vi "Real Moving Average testing.vi"() -> ()   [LabVIEW 2009]
panel:
  out "Waveform Graph":cluster{"Average Array":dbl[]}[](graph)
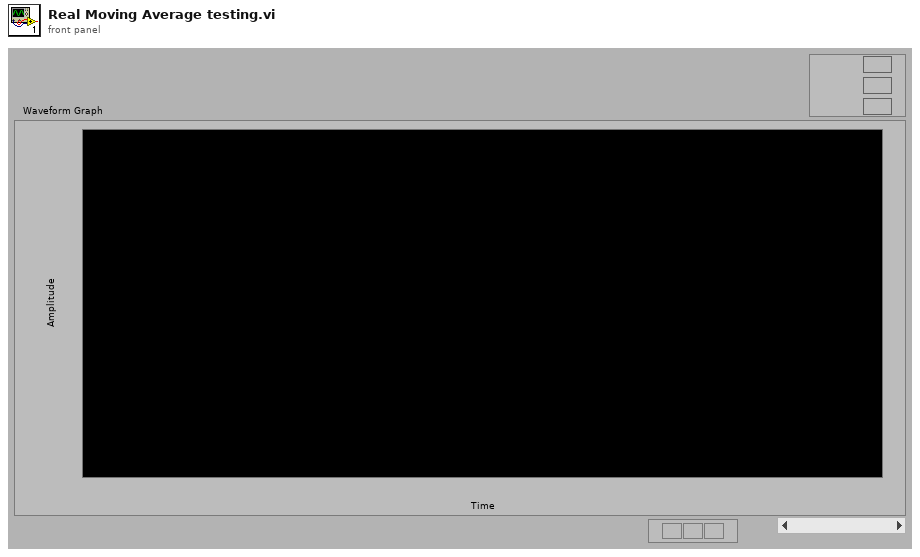
[diagram p1: front panel]
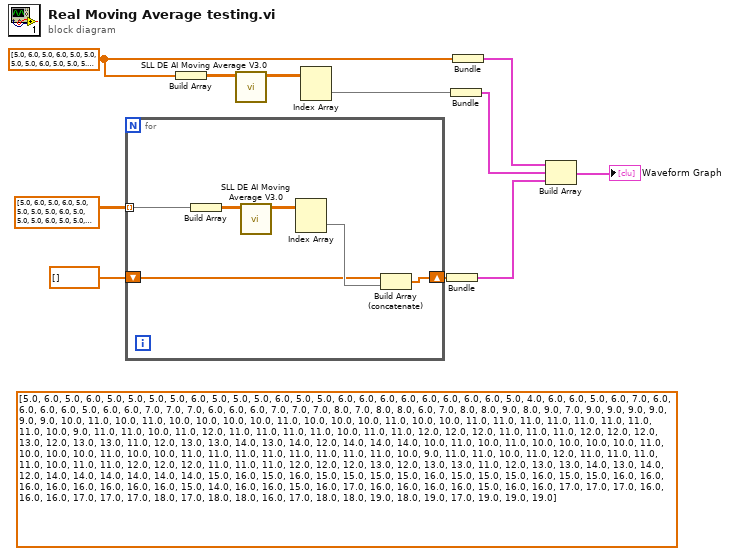
[diagram p0: block diagram]
diagram:
  (unwired) dbl[][] [[5.0, 6.0, 5.0, 6.0, 5.0, 5.0, 5.0, 5.0, 6.0, 5.0, 5.0, 5.0, 6.0, 5.0, 5.0, 6.0, 6.0, 6.0, 6.0, 6.0, 6.0, 6.0, 6.0, 5.0, 4.0, 6.0, 6.0, 5.0, 6.0, 7.0, 6.0, 6.0, 6.0, 6.0, 5.0, 6.0, 6.0, 7.0, 7.0, 7.0, 6.0, 6.0, 6.0, 7.0, 7.0, 7.0, 8.0, 7.0, 8.0, 8.0], [6.0, 7.0, 8.0, 8.0, 9.0, 8.0, 9.0, 7.0, 9.0, 9.0, 9.0, 9.0, 9.0, 9.0, 10.0, 11.0, 10.0, 11.0, 10.0, 10.0, 10.0, 10.0, 11.0, 10.0, 10.0, 10.0, 11.0, 10.0, 10.0, 11.0, 11.0, 11.0, 11.0, 11.0, 11.0, 11.0, 11.0, 10.0, 9.0, 11.0, 11.0, 10.0, 11.0, 12.0, 11.0, 11.0, 11.0, 11.0, 10.0, 11.0], [11.0, 12.0, 12.0, 12.0, 11.0, 11.0, 11.0, 12.0, 12.0, 12.0, 13.0, 12.0, 13.0, 13.0, 11.0, 12.0, 13.0, 13.0, 14.0, 13.0, 14.0, 12.0, 14.0, 14.0, 14.0, 10.0, 11.0, 10.0, 11.0, 10.0, 10.0, 10.0, 10.0, 11.0, 10.0, 10.0, 10.0, 11.0, 10.0, 10.0, 11.0, 11.0, 11.0, 11.0, 11.0, 11.0, 11.0, 11.0, 10.0, 9.0], [11.0, 11.0, 10.0, 11.0, 12.0, 11.0, 11.0, 11.0, 11.0, 10.0, 11.0, 11.0, 12.0, 12.0, 12.0, 11.0, 11.0, 11.0, 12.0, 12.0, 12.0, 13.0, 12.0, 13.0, 13.0, 11.0, 12.0, 13.0, 13.0, 14.0, 13.0, 14.0, 12.0, 14.0, 14.0, 14.0, 14.0, 14.0, 14.0, 15.0, 16.0, 15.0, 16.0, 15.0, 15.0, 15.0, 15.0, 16.0, 15.0, 15.0], [15.0, 16.0, 15.0, 15.0, 16.0, 16.0, 16.0, 16.0, 16.0, 16.0, 16.0, 16.0, 15.0, 14.0, 16.0, 16.0, 15.0, 16.0, 17.0, 16.0, 16.0, 16.0, 16.0, 15.0, 16.0, 16.0, 17.0, 17.0, 17.0, 16.0, 16.0, 16.0, 17.0, 17.0, 17.0, 18.0, 17.0, 18.0, 18.0, 16.0, 17.0, 18.0, 18.0, 19.0, 18.0, 19.0, 17.0, 19.0, 19.0, 19.0]] ("Array")
  w4 = dbl[] [5.0, 6.0, 5.0, 6.0, 5.0, 5.0, 5.0, 5.0, 6.0, 5.0, 5.0, 5.0, 6.0, 5.0, 5.0, 6.0, 6.0, 6.0, 6.0, 6.0, 6.0, 6.0, 6.0, 5.0, 4.0, 6.0, 6.0, 5.0, 6.0, 7.0, 6.0, 6.0, 6.0, 6.0, 5.0, 6.0, 6.0, 7.0, 7.0, 7.0, 6.0, 6.0, 6.0, 7.0, 7.0, 7.0, 8.0, 7.0, 8.0, 8.0, 6.0, 7.0, 8.0, 8.0, 9.0, 8.0, 9.0, 7.0, 9.0, 9.0, 9.0, 9.0, 9.0, 9.0, 10.0, 11.0, 10.0, 11.0, 10.0, 10.0, 10.0, 10.0, 11.0, 10.0, 10.0, 10.0, 11.0, 10.0, 10.0, 11.0, 11.0, 11.0, 11.0, 11.0, 11.0, 11.0, 11.0, 10.0, 9.0, 11.0, 11.0, 10.0, 11.0, 12.0, 11.0, 11.0, 11.0, 11.0, 10.0, 11.0, 11.0, 12.0, 12.0, 12.0, 11.0, 11.0, 11.0, 12.0, 12.0, 12.0, 13.0, 12.0, 13.0, 13.0, 11.0, 12.0, 13.0, 13.0, 14.0, 13.0, 14.0, 12.0, 14.0, 14.0, 14.0, 10.0, 11.0, 10.0, 11.0, 10.0, 10.0, 10.0, 10.0, 11.0, 10.0, 10.0, 10.0, 11.0, 10.0, 10.0, 11.0, 11.0, 11.0, 11.0, 11.0, 11.0, 11.0, 11.0, 10.0, 9.0, 11.0, 11.0, 10.0, 11.0, 12.0, 11.0, 11.0, 11.0, 11.0, 10.0, 11.0, 11.0, 12.0, 12.0, 12.0, 11.0, 11.0, 11.0, 12.0, 12.0, 12.0, 13.0, 12.0, 13.0, 13.0, 11.0, 12.0, 13.0, 13.0, 14.0, 13.0, 14.0, 12.0, 14.0, 14.0, 14.0, 14.0, 14.0, 14.0, 15.0, 16.0, 15.0, 16.0, 15.0, 15.0, 15.0, 15.0, 16.0, 15.0, 15.0, 15.0, 16.0, 15.0, 15.0, 16.0, 16.0, 16.0, 16.0, 16.0, 16.0, 16.0, 16.0, 15.0, 14.0, 16.0, 16.0, 15.0, 16.0, 17.0, 16.0, 16.0, 16.0, 16.0, 15.0, 16.0, 16.0, 17.0, 17.0, 17.0, 16.0, 16.0, 16.0, 17.0, 17.0, 17.0, 18.0, 17.0, 18.0, 18.0, 16.0, 17.0, 18.0, 18.0, 19.0, 18.0, 19.0, 17.0, 19.0, 19.0, 19.0] ("x+y")
  n1 = for {
    tunnel: dbl[][] [[5.0, 6.0, 5.0, 6.0, 5.0, 5.0, 5.0, 5.0, 6.0, 5.0, 5.0, 5.0, 6.0, 5.0, 5.0, 6.0, 6.0, 6.0, 6.0, 6.0, 6.0, 6.0, 6.0, 5.0, 4.0, 6.0, 6.0, 5.0, 6.0, 7.0, 6.0, 6.0, 6.0, 6.0, 5.0, 6.0, 6.0, 7.0, 7.0, 7.0, 6.0, 6.0, 6.0, 7.0, 7.0, 7.0, 8.0, 7.0, 8.0, 8.0], [6.0, 7.0, 8.0, 8.0, 9.0, 8.0, 9.0, 7.0, 9.0, 9.0, 9.0, 9.0, 9.0, 9.0, 10.0, 11.0, 10.0, 11.0, 10.0, 10.0, 10.0, 10.0, 11.0, 10.0, 10.0, 10.0, 11.0, 10.0, 10.0, 11.0, 11.0, 11.0, 11.0, 11.0, 11.0, 11.0, 11.0, 10.0, 9.0, 11.0, 11.0, 10.0, 11.0, 12.0, 11.0, 11.0, 11.0, 11.0, 10.0, 11.0], [11.0, 12.0, 12.0, 12.0, 11.0, 11.0, 11.0, 12.0, 12.0, 12.0, 13.0, 12.0, 13.0, 13.0, 11.0, 12.0, 13.0, 13.0, 14.0, 13.0, 14.0, 12.0, 14.0, 14.0, 14.0, 10.0, 11.0, 10.0, 11.0, 10.0, 10.0, 10.0, 10.0, 11.0, 10.0, 10.0, 10.0, 11.0, 10.0, 10.0, 11.0, 11.0, 11.0, 11.0, 11.0, 11.0, 11.0, 11.0, 10.0, 9.0], [11.0, 11.0, 10.0, 11.0, 12.0, 11.0, 11.0, 11.0, 11.0, 10.0, 11.0, 11.0, 12.0, 12.0, 12.0, 11.0, 11.0, 11.0, 12.0, 12.0, 12.0, 13.0, 12.0, 13.0, 13.0, 11.0, 12.0, 13.0, 13.0, 14.0, 13.0, 14.0, 12.0, 14.0, 14.0, 14.0, 14.0, 14.0, 14.0, 15.0, 16.0, 15.0, 16.0, 15.0, 15.0, 15.0, 15.0, 16.0, 15.0, 15.0], [15.0, 16.0, 15.0, 15.0, 16.0, 16.0, 16.0, 16.0, 16.0, 16.0, 16.0, 16.0, 15.0, 14.0, 16.0, 16.0, 15.0, 16.0, 17.0, 16.0, 16.0, 16.0, 16.0, 15.0, 16.0, 16.0, 17.0, 17.0, 17.0, 16.0, 16.0, 16.0, 17.0, 17.0, 17.0, 18.0, 17.0, 18.0, 18.0, 16.0, 17.0, 18.0, 18.0, 19.0, 18.0, 19.0, 17.0, 19.0, 19.0, 19.0]] ("Array") -> [w17] mode=indexing
    shift-right: [w15] -> w10
    shift-left: dbl[] [] -> [w14]
    n2 = Build Array(w17) -> (w12:dbl[][])
    n3 = call "SLL DE AI Moving Average V3.0.vi"("Input Array"=w12) -> ("Averaged Array"=w13:dbl[][])  [unwired: 9 in, 1 out]
    n4 = Index Array(array=w13) -> (element=w16:dbl[])  [unwired: 2 in]
    n5 = Build Array (concatenate)(w14, w16) -> (w15:dbl[])
  }
  n6 = Build Array(w4) -> (w7:dbl[][])
  n7 = call "SLL DE AI Moving Average V3.0.vi"("Input Array"=w7) -> ("Averaged Array"=w6:dbl[][])  [unwired: 9 in, 1 out]
  n8 = Index Array(array=w6) -> (element=w5:dbl[])  [unwired: 2 in]
  n9 = Bundle(w10) -> (w2:cluster{dbl[]})  [unwired: 1 in]
  n10 = Bundle("Averaged Array"=w5) -> (w1:cluster{"Averaged Array":dbl[]})  [unwired: 1 in]
  n11 = Bundle("x+y"=w4) -> (w8:cluster{"x+y":dbl[]})  [unwired: 1 in]
  n12 = Build Array(w8, w1, w2) -> (→"Waveform Graph":cluster{"Averaged Array":dbl[]}[])
